vi "Numeric-to-String-to-Numeric.vi"() -> ()   [LabVIEW 2016]
panel:
  out "String-to-number":dbl
  out "F-format string":string
  in  "number":dbl
  in  "width (-)":i16
  in  "precision (6)":i16
  in  "use system decimal point (T)":bool
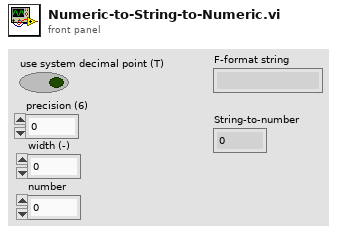
[diagram p1: front panel]
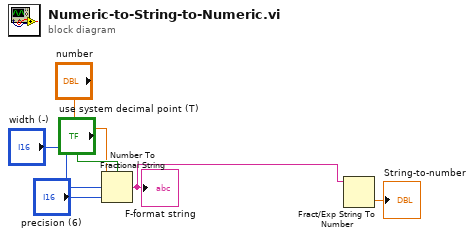
[diagram p0: block diagram]
diagram:
  n1 = Number To Fractional String(use system decimal point (T)="use system decimal point (T)", number="number", width (-)="width (-)", precision (6)="precision (6)") -> (F-format string=w2:string)
  "F-format string" <- w2
  n2 = Fract/Exp String To Number(string=w2) -> (number=→"String-to-number":dbl)  [unwired: 3 in, 1 out]
